vi "Cycle 0 Pass-Fail and Report Text.vi"(0 "Drive Cycle State":T1 {"ERD Number" format="%.0x"}, 5 "Motor Mode":T1 {"ERD Number" format="%.0x"}, 7 "Previous Pass/Fail":bool, 9 "Cycle State Expected":string, 11 "Motor Mode Expected":string, 13 "Header":string) -> (8 "Pass/Fail?":bool, 10 "Report Text":string)   [LabVIEW 2016, in "TL27.lvlib"]
uses:
  Projects/TL27.lvlib
  Common/LabVIEW GEA2 Toolkit/LabVIEW_GEA2_Toolkit.lvlibp/type defs/ERD Read Data Out.ctl
  Common/LabVIEW GEA2 Toolkit/LabVIEW_GEA2_Toolkit.lvlibp
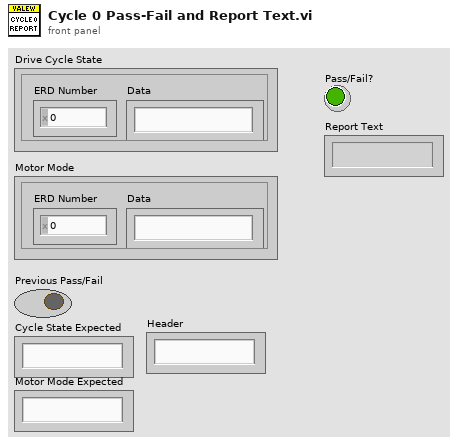
[diagram p1: front panel]
types:
  T1 = typedef "LabVIEW_GEA2_Toolkit.lvlibp/ERD Read Data Out.ctl" = cluster{"ERD Number":u16, "Data":string}
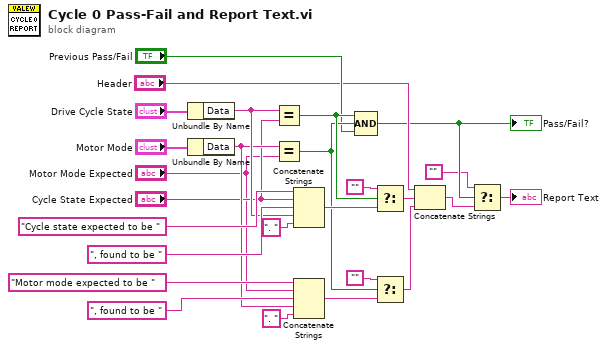
[diagram p0: block diagram]
diagram:
  n1 = Unbundle By Name("Drive Cycle State") -> ("Data"=w20:string)
  n2 = Unbundle By Name("Motor Mode") -> ("Data"=w11:string)
  n3 = Equal?(x=w20, y="Cycle State Expected") -> (x = y?=w25:bool)
  n4 = Equal?(x=w11, y="Motor Mode Expected") -> (x = y?=w12:bool)
  n5 = Concatenate Strings("Cycle state expected to be " ("string"), "Cycle State Expected", ", found to be " ("string"), w20, ". " ("string")) -> (w26:string)
  n6 = Concatenate Strings("Motor mode expected to be " ("string"), "Motor Mode Expected", ", found to be " ("string"), w11, ". " ("string")) -> (w14:string)
  n7 = Compound Arithmetic op=AND(w25, w12, "Previous Pass/Fail") -> (w3:bool)
  "Pass/Fail?" <- w3
  n8 = Select(t="", s=w25, f=w26) -> (s? t:f=w23:string)
  n9 = Select(t="", s=w12, f=w14) -> (s? t:f=w13:string)
  n10 = Concatenate Strings("Header", w23, w13) -> (w2:string)
  n11 = Select(t="", s=w3, f=w2) -> (s? t:f=→"Report Text":string)
